vi "Door2.vi"(0 "Strings in":string[](array[string])=["C:\\CuspControl\\GPIB and Network\\Cusp\\Dummyfile.txt", "6723"], 1 "Dubs in":dbl[](array[numeric])=[0.0]) -> ()   [LabVIEW 2018]
uses:
  <vilib>/Analysis/1siggen.llb/Ramp Pattern by Samples.vi
  <vilib>/DAQmx/write.llb/DAQmx Write (Analog 1D DBL 1Chan NSamp).vi
  <vilib>/DAQmx/create/channels.llb/DAQmx Create Channel (AO-Voltage-Basic).vi
  <vilib>/DAQmx/configure/timing.llb/DAQmx Timing (Sample Clock).vi
  <vilib>/DAQmx/miscellaneous.llb/DAQmx Fill In Error Info.vi
  <vilib>/Analysis/NI_AALBase.lvlib
panel:
  in  "rate":dbl=1000.0 format="%0.2f"
  out "Ramp Pattern":dbl[](array[numeric])
  in  "samples":i32=128
  in  "file (use dialog)":path=path "C:/CuspControl/GPIB and Network/Cusp/DoorVolts.txt"
  in  "subvi":bool=TRUE
  out "error out":errorcluster
  in  "AO2 name":string="6723"
  in  "Takasago Vc ao line":string="/ao12"
  in  "ON voltage":dbl format="%#_13g"
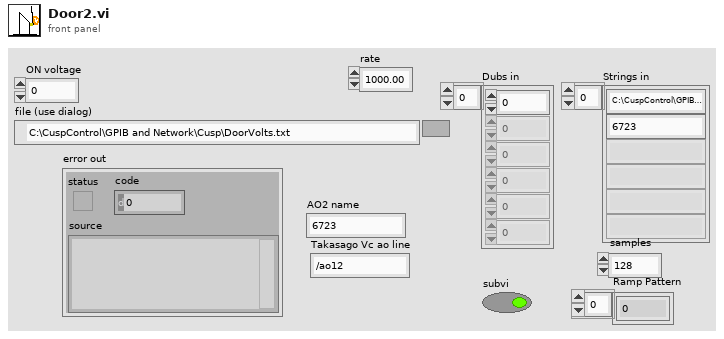
[diagram p1: front panel]
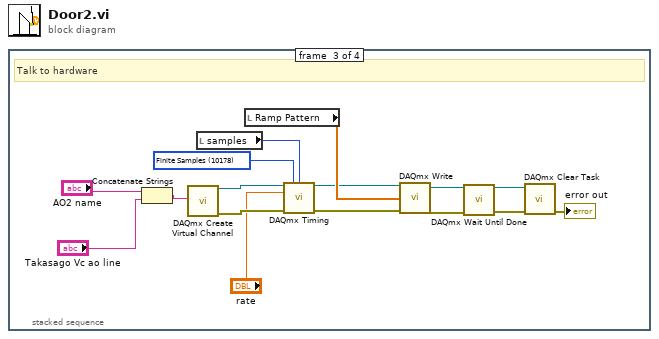
[diagram p0: block diagram]
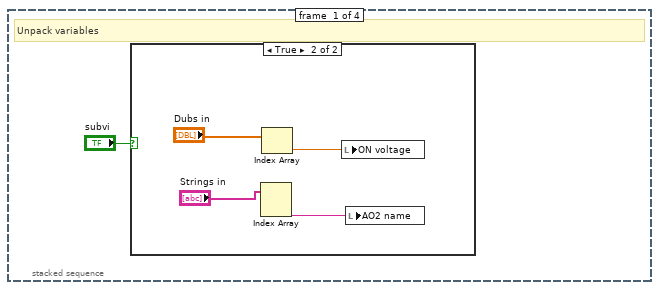
[diagram p2: hidden frame]
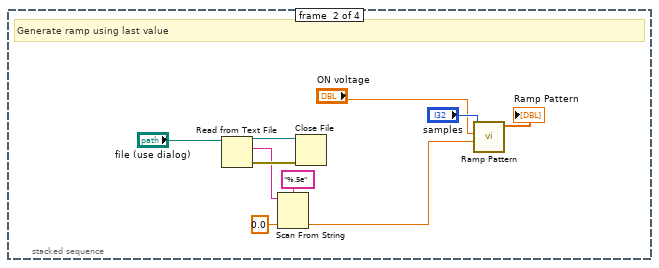
[diagram p4: hidden frame]
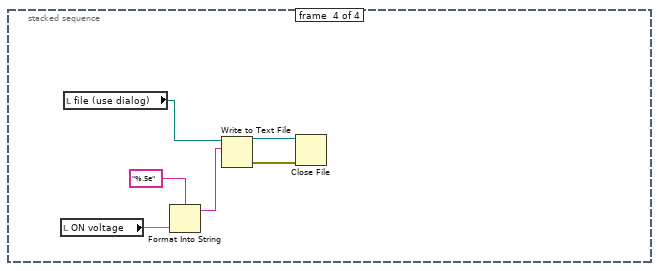
[diagram p5: hidden frame]
diagram:
  n1 = stacked-sequence {
    frame #0 {
      # "Unpack variables"
      n2 = case shown="True" "subvi" {
        frame False {
        }
        frame True {
          n3 = Index Array(array="Strings in") -> (element #2=w2:string)  [unwired: 2 in, 1 out]
          n4 = Index Array(array="Dubs in") -> (element=w3:dbl)  [unwired: 1 in]
          n5 = local write "ON voltage"(w3) -> ()
          n6 = local write "AO2 name"(w2) -> ()
        }
      }
    }
    frame #1 {
      # "Generate ramp using last value"
      n7 = Read from Text File(file (use dialog)="file (use dialog)") -> (refnum out=w10:refnum<file>, text=w8:string, error out=w9:errorcluster)  [unwired: 3 in, 1 out]
      n8 = Scan From String(format string="%.5e", input string=w8, default 1=0.0 ("default value 1")) -> (output 1=w15:dbl)  [unwired: 2 in, 3 out]
      n9 = Close File(refnum=w10, error in=w9) -> ()  [unwired: 2 out]
      n10 = call-poly <vilib>:"Ramp Pattern.vi"("start"=w15, "end"="ON voltage", "samples"="samples") -> ("Ramp Pattern"=→"Ramp Pattern":dbl[])  [unwired: 7 in, 1 out]
    }
    frame #2 {
      w17 = 10178 items=["Finite Samples"=10178, "Continuous Samples"=10123, "Hardware Timed Single Point"=12522] ("sample mode")
      # "Talk to hardware"
      n11 = Concatenate Strings("AO2 name", "Takasago Vc ao line") -> (w27:string)
      n12 = call-poly <vilib>:"DAQmx Create Virtual Channel.vi"("physical channels"=w27) -> ("task out"=w22:refnum<k21>, "error out"=w21:errorcluster)  [unwired: 13 in]
      n13 = local read "samples"() -> (w18:i32)
      n14 = local read "Ramp Pattern"() -> (w23:dbl[])
      n15 = call-poly <vilib>:"DAQmx Timing.vi"("task/channels in"=w22, "sample mode"=w17, "samples per channel"=w18, "rate"="rate", "error in"=w21) -> ("task out"=w19:refnum<k21>, "error out"=w20:errorcluster)  [unwired: 9 in]
      n16 = call-poly <vilib>:"DAQmx Write.vi"("task/channels in"=w19, "data"=w23, "error in"=w20) -> ("task out"=w29:refnum<k21>, "error out"=w28:errorcluster)  [unwired: 10 in, 1 out]
      n17 = call <vilib>:"DAQmx Wait Until Done.vi"("task/channels in"=w29, "error in"=w28) -> ("task out"=w31:refnum<k21>, "error out"=w30:errorcluster)  [unwired: 12 in]
      n18 = call <vilib>:"DAQmx Clear Task.vi"("task in"=w31, "error in"=w30) -> ("error out"=→"error out":errorcluster)  [unwired: 13 in]
    }
    frame #3 {
      n19 = local read "ON voltage"() -> (w34:dbl)
      n20 = local read "file (use dialog)"() -> (w35:path)
      n21 = Format Into String(format string="%.5e", w34) -> (resulting string=w33:string)  [unwired: 2 in, 1 out]
      n22 = Write to Text File(file (use dialog)=w35, text=w33) -> (refnum out=w37:refnum<file>, error out=w36:errorcluster)  [unwired: 2 in, 1 out]
      n23 = Close File(refnum=w37, error in=w36) -> ()  [unwired: 2 out]
    }
  }
